vi "Module Loop.vi"(8 "error in (no error)":errorcluster, 11 "GenericGuiDI in":refnum<class "GenericGuiDI.lvclass">) -> (0 "error out":errorcluster, 3 "GenericGuiDI out":refnum<class "GenericGuiDI.lvclass">)   [LabVIEW 2020, in "VolatusDAQGenericGUI.lvlib" / "GenericGuiDI.lvclass"]
uses:
  GenericGuiDI.lvclass
  C:/dev/lv20CE/relink/lv-volatus/Volatus/Module/Module.lvclass
  Volatus/Module/Module.lvclass/Module.ctl
  Volatus/MessageQ/MessageQ.lvclass/MessageQ.ctl
  GenericGuiDI.lvclass/GenericGuiDI.ctl
  Volatus/Module/Module.lvclass
  <vilib>/Utility/error.llb/Error Cluster From Error Code.vi
  Volatus/MessageQ/MessageQ.lvclass
  VolatusDAQGenericGUI.lvlib
  Volatus/VolatusAPI/VolatusAPI.lvclass
  VolatusGUI/GUI Helper/GUI Helper.lvclass
panel:
  in  "Tree":string(tree)
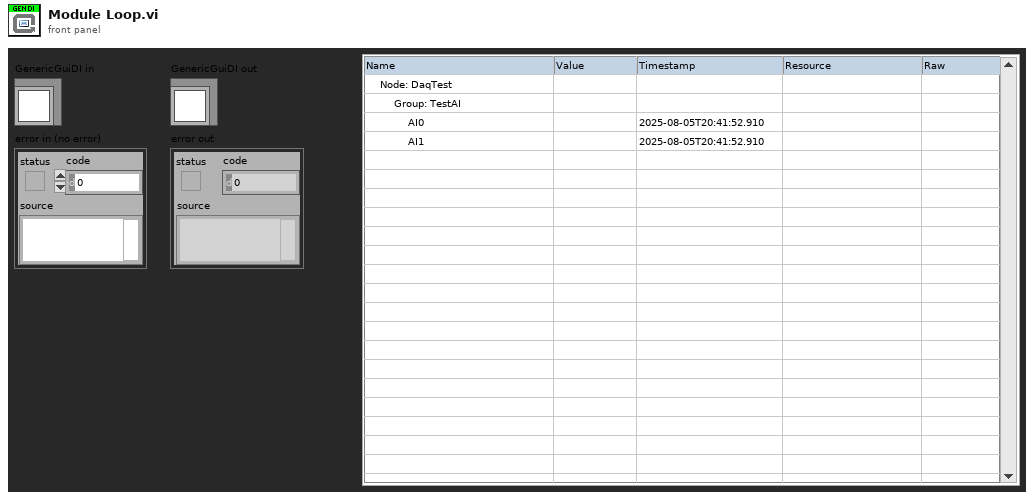
[diagram p1: front panel]
types:
  T1 = enum32{"Invalid", "Standard", "Closed", "Hidden", "Minimized", "Maximized"}
  T2 = typedef "VolatusDAQGenericGUI.lvlib/Group Info.ctl" = cluster{"Group":refnum<class "Group.lvclass">, "Channel Names":string[], "Resources":string[], "Node":string, "Task":string}
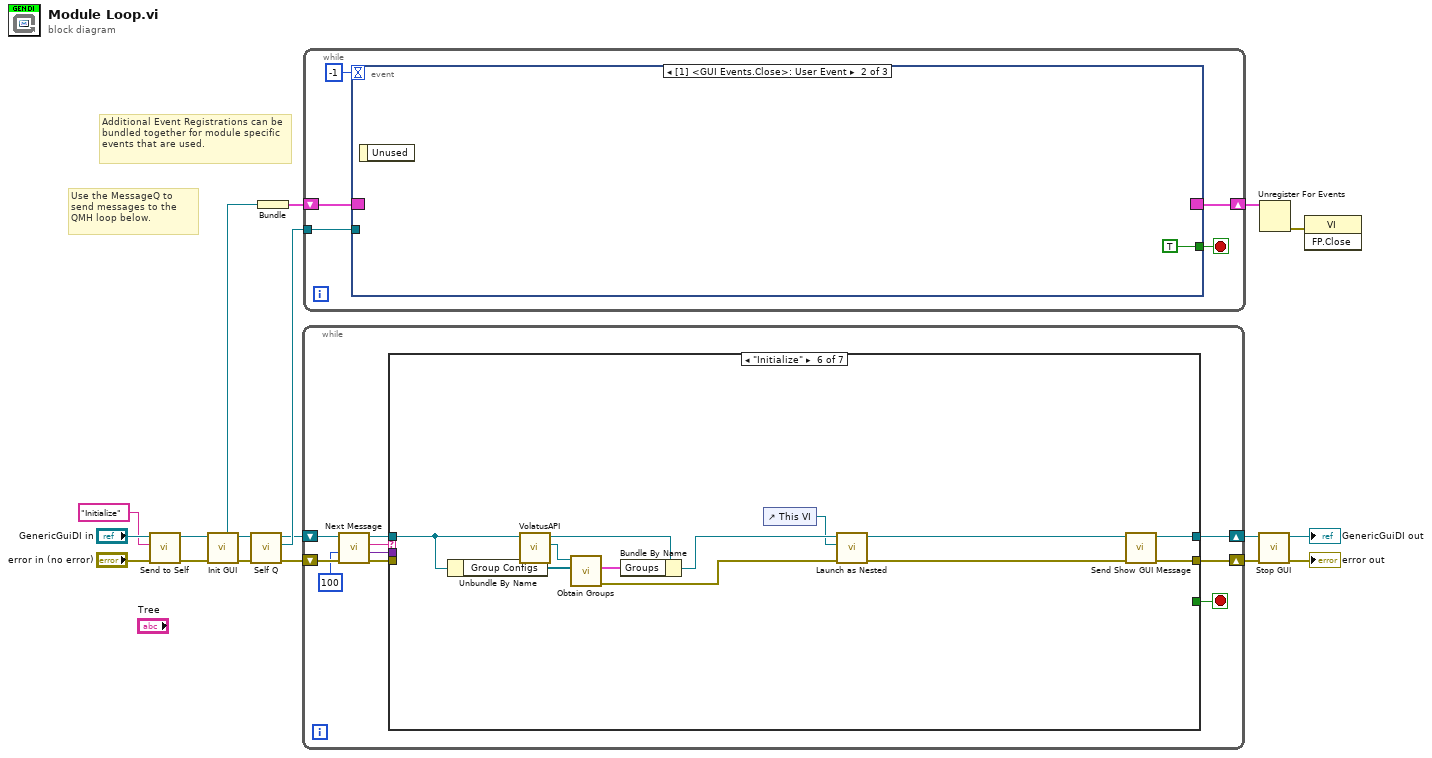
[diagram p0: block diagram]
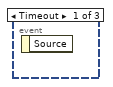
[diagram p2: hidden frame]
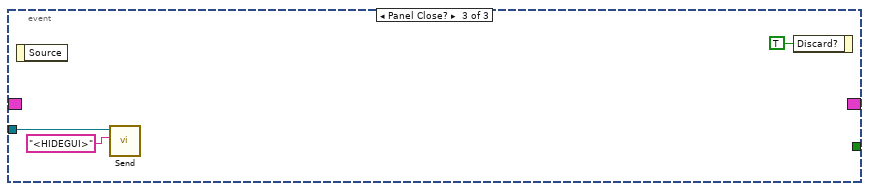
[diagram p3: hidden frame]
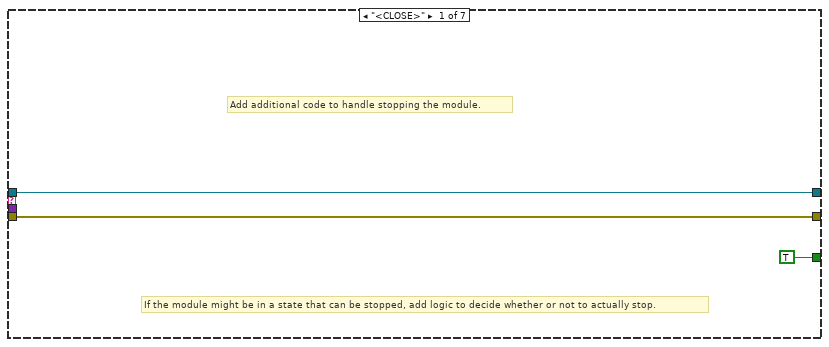
[diagram p4: hidden frame]
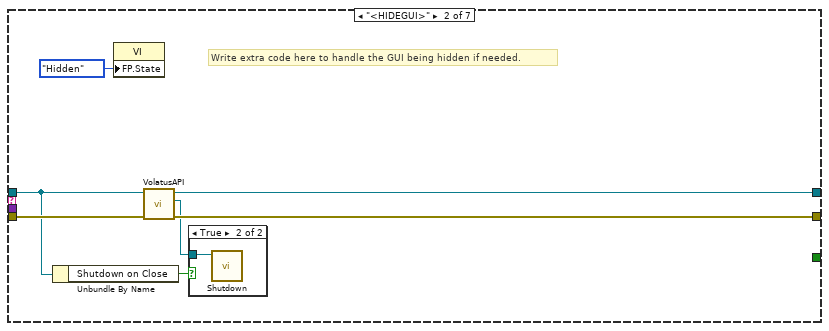
[diagram p5: hidden frame]
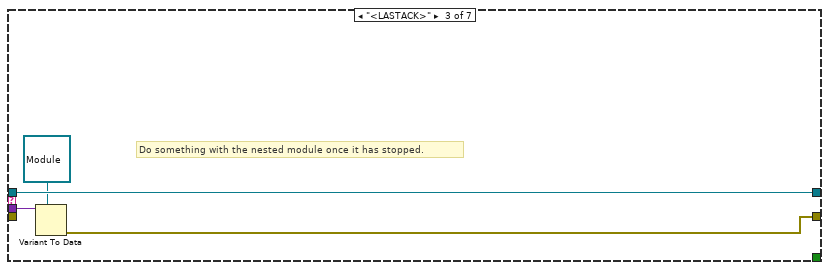
[diagram p7: hidden frame]
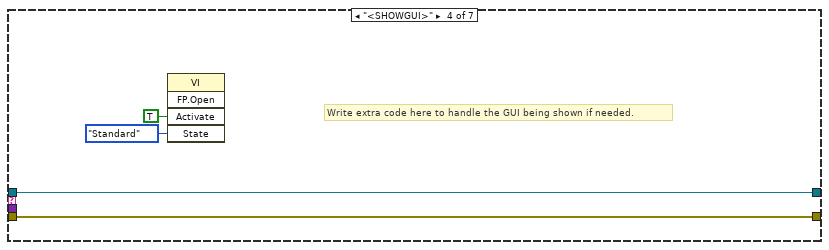
[diagram p8: hidden frame]
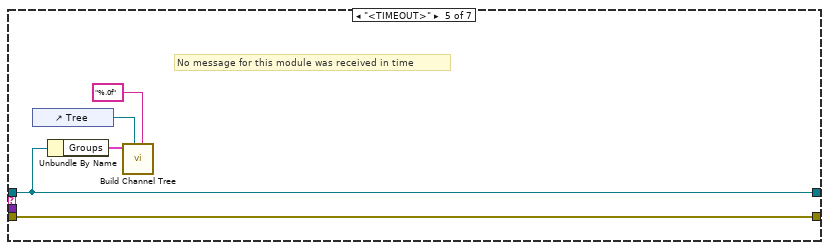
[diagram p9: hidden frame]
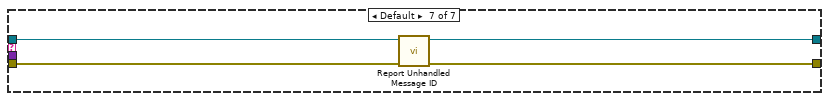
[diagram p10: hidden frame]
diagram:
  # "Additional Event Registrations can be bundled together for module specific events that are used."
  # "Use the MessageQ to send messages to the QMH loop below."
  n1 = call "Send to Self.vi"("error in (no error)"="error in (no error)", "Message ID"="Initialize", "Module in"="GenericGuiDI in") -> ("error out"=w4:errorcluster, "Module out"=w2:refnum<class "GenericGuiDI.lvclass">)  [unwired: 7 in]
  n2 = call "Init GUI.vi"("Module in"=w2) -> ("Module out"=w10:refnum<class "GenericGuiDI.lvclass">, "Event Reg"=w15:refnum<event-registration>)  [unwired: 9 in]
  n3 = call "Self Q.vi"("Module in"=w10) -> ("Self Q"=w9:refnum<class "MessageQ.lvclass">, "Module out"=w8:refnum<class "GenericGuiDI.lvclass">)  [unwired: 9 in]
  n4 = Bundle("Event Reg"=w15) -> (w11:cluster{"Event Reg":refnum<event-registration>})  [unwired: 1 in]
  n5 = while {
    shift-right: [w21] -> w13
    shift-left: w8 -> [w26]
    shift-right: [w20] -> w14
    shift-left: w4 -> [w25]
    stop <- w19 stop-if-true
    n6 = call "Next Message.vi"("error in (no error)"=w25, "Timeout ms (-1)"=100, "Module in"=w26) -> ("error out"=w24:errorcluster, "Data"=w18:variant, "ID"=w23:string, "Module out"=w22:refnum<class "GenericGuiDI.lvclass">)  [unwired: 5 in]
    n7 = case shown="\"Initialize\"" w23 {
      tunnel: w24 -> [w27 w35 _ w43 w49 _ w65]
      tunnel: w22 -> [w28 w30 w40 w44 w48 w57 w63]
      tunnel: [w28 w31 w40 w44 w48 w54 w62] -> w21
      tunnel: [w27 w35 w37 w43 w49 w55 w64] -> w20
      tunnel: [TRUE _ _ _ _ _ _] -> w19
      tunnel: w18 -> [_ _ w39 _ _ _ _]
      frame "<CLOSE>" {
        # "If the module might be in a state that can be stopped, add logic to decide whether or not to actually stop."
        # "Add additional code to handle stopping the module."
      }
      frame "<HIDEGUI>" {
        # "Write extra code here to handle the GUI being hidden if needed."
        n8 = Unbundle By Name(w30) -> ("Shutdown on Close"=w33:bool)
        n9 = property class="VI"("FP.State"=T1."Hidden" ("Front Panel Window:State")) -> ()  [unwired: 2 in, 2 out]
        n10 = call "VolatusAPI.vi"("Module in"=w30) -> ("VolatusAPI"=w32:refnum<class "VolatusAPI.lvclass">, "Module out"=w31:refnum<class "GenericGuiDI.lvclass">)  [unwired: 9 in]
        n11 = case shown="True" w33 {
          tunnel: w32 -> [_ w36]
          frame False {
          }
          frame True {
            n12 = call "Shutdown.vi"("VolatusAPI in"=w36) -> ()  [unwired: 9 in, 2 out]
          }
        }
      }
      frame "<LASTACK>" {
        # "Do something with the nested module once it has stopped."
        n13 = Variant To Data(type=refnum<class "Module.lvclass"> refnum ("Volatus:Module"), Variant=w39) -> (error out=w37:errorcluster)  [unwired: 1 in, 1 out]
      }
      frame "<SHOWGUI>" {
        # "Write extra code here to handle the GUI being shown if needed."
        n14 = invoke class="VI" method="FP.Open"("Activate"=TRUE ("Activate?"), "State"=T1."Standard") -> ()  [unwired: 3 in, 5 out]
      }
      frame "<TIMEOUT>" {
        # "No message for this module was received in time"
        n15 = control-ref of="Tree"() -> (w46:refnum<vi>)
        n16 = Unbundle By Name(w48) -> ("Groups"=w47:T2[])
        n17 = call "Build Channel Tree.vi"("Value Format"="%.0f", "Tree"=w46, "Groups"=w47) -> ()  [unwired: 9 in]
      }
      frame "Initialize" {
        n18 = Unbundle By Name(w57) -> ("Group Configs"=w60:refnum<class "Group.lvclass">[])
        n19 = call "VolatusAPI.vi"("Module in"=w57) -> ("VolatusAPI"=w59:refnum<class "VolatusAPI.lvclass">, "Module out"=w61:refnum<class "GenericGuiDI.lvclass">)  [unwired: 9 in]
        n20 = call "Obtain Groups.vi"("Group Configs"=w60, "VolatusAPI"=w59) -> ("error out"=w56:errorcluster, "Groups"=w58:T2[])  [unwired: 8 in]
        n21 = Bundle By Name(cluster=w61, "Groups"=w58) -> (w51:refnum<class "GenericGuiDI.lvclass">)
        n22 = control-ref of="This VI"() -> (w50:refnum<vi>)
        n23 = call "Launch as Nested.vi"("error in (no error)"=w56, "GUI"=w50, "Parent in"=w51) -> ("error out"=w53:errorcluster, "Parent"=w52:refnum<class "GenericGuiDI.lvclass">)  [unwired: 6 in, 1 out]
        n24 = call "Send Show GUI Message.vi"("error in (no error)"=w53, "Module in"=w52) -> ("error out"=w55:errorcluster, "Module out"=w54:refnum<class "GenericGuiDI.lvclass">)  [unwired: 8 in]
      }
      frame Default {
        n25 = call "Report Unhandled Message ID.vi"("error in (no error)"=w65, "Module in"=w63) -> ("error out"=w64:errorcluster, "Module out"=w62:refnum<class "GenericGuiDI.lvclass">)  [unwired: 8 in]
      }
    }
  }
  n26 = while {
    tunnel: w9 -> [w70]
    shift-right: [w68] -> w12
    shift-left: w11 -> [w69]
    stop <- w67 stop-if-true
    n27 = event shown="[1] <GUI Events.Close>: User Event" {
      selector: w69 -> [_ _ _]
      dyn-events: [_ _ _] -> w68
      timeout: -1 -> [_ _ _]
      tunnel: w70 -> [_ _ w73]
      tunnel: [_ TRUE _] -> w67
      event Timeout {
        n28 = event-data() -> ()  [unwired: 1 in, 1 out]
      }
      event User Event {
        n29 = event-data() -> ()  [unwired: 1 in, 1 out]
      }
      event Panel Close? {
        n30 = event-data() -> ()  [unwired: 1 in, 1 out]
        n31 = call "Send.vi"("ID"="<HIDEGUI>", "MessageQ in"=w73) -> ()  [unwired: 8 in, 2 out]
        n32 = event-data("Discard?"=TRUE) -> ()  [unwired: 1 in, 1 out]
      }
    }
  }
  n33 = call "Stop GUI.vi"("error in (no error)"=w14, "Module in"=w13) -> ("error out"=→"error out":errorcluster, "Module out"=→"GenericGuiDI out":refnum<class "GenericGuiDI.lvclass">)  [unwired: 8 in]
  n34 = Unregister For Events(event registration refnum=w12) -> (error out=w16:errorcluster)  [unwired: 1 in]
  n35 = invoke class="VI" method="FP.Close"(error in=w16) -> ()  [unwired: 2 in, 3 out]
